vi "Choreo_ReadTrajectoryFile_Example.vi"(11 "Trajectory File Name":path=path "../Deploy/ChoreoTrajectory") -> (0 "error out":errorcluster)   [LabVIEW 2019]
uses:
  <vilib>/Rock Robotics/WPI/ThirdParty/ChoreoLib/TypeDef/ChoreoTrajectorySwerve.ctl
  <vilib>/Rock Robotics/WPI/ThirdParty/ChoreoLib/TypeDef/ChoreoSwerveSample.ctl
  <vilib>/Rock Robotics/WPI/ThirdParty/ChoreoLib/TypeDef/ChoreoEventMarker.ctl
  <vilib>/Rock Robotics/WPI/ThirdParty/ChoreoLib/ChoreoLib.lvlib
panel:
  out "ChoreoTrajectorySwerve":T1
  in  "Read File":bool
  # "Relative or absolute trajectory\nfile name"
  # "NOTE:  For relative trajectory file names, \nthe file must be copied to the \n\n        Documents\\LabVIEW Data\\choreo \n\ndirectory."
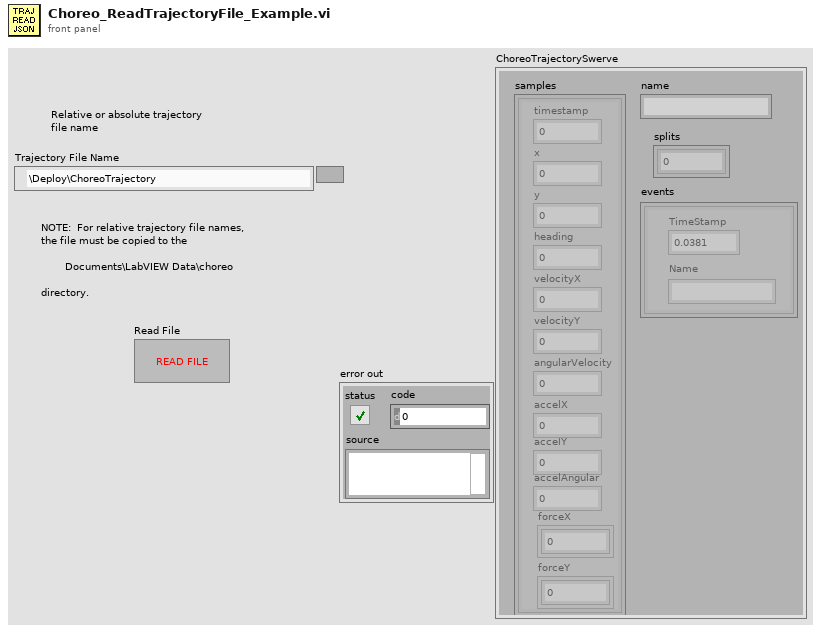
[diagram p1: front panel]
types:
  T1 = typedef "ChoreoLib.lvlib/ChoreoTrajectorySwerve.ctl" = cluster{"name":string, "samples":T2[], "splits":i32[], "events":T3[]}
  T2 = typedef "ChoreoLib.lvlib/ChoreoSwerveSample.ctl" = cluster{"timestamp":dbl, "x":dbl, "y":dbl, "heading":dbl, "velocityX":dbl, "velocityY":dbl, "angularVelocity":dbl, "accelX":dbl, "accelY":dbl, "accelAngular":dbl, "forceX":dbl[], "forceY":dbl[]}
  T3 = typedef "ChoreoLib.lvlib/ChoreoEventMarker.ctl" = cluster{"TimeStamp":dbl, "Name":string}
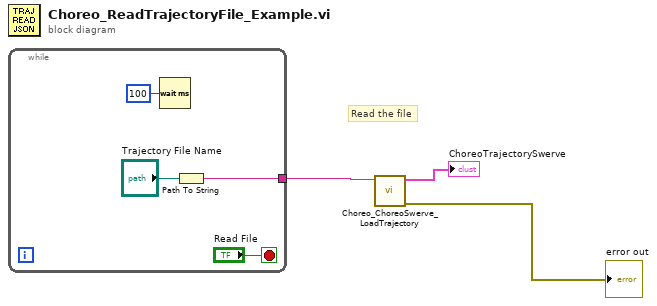
[diagram p0: block diagram]
diagram:
  # "Read the file"
  n1 = while {
    tunnel: [w6] -> w3
    stop <- "Read File" stop-if-true
    n2 = Wait (ms)(milliseconds to wait=u32 100) -> ()  [unwired: 1 out]
    n3 = Path To String(path="Trajectory File Name") -> (string=w6:string)
  }
  n4 = call <vilib>:"Choreo_ChoreoSwerve_LoadTrajectory.vi"("FileName"=w3) -> ("error out"=→"error out":errorcluster, "ChoreoTrajectorySwerve"=→"ChoreoTrajectorySwerve":T1)  [unwired: 8 in, 1 out]
